vi "Configure Smoothing.vi"(7 "Enable Calculate1 (T: Enable)":bool=TRUE, 8 "error in (no error)":errorcluster, 9 "Enable Smoothing (T: Enable)":bool=TRUE, 10 "Measurement Number (2: Fast)":i32(ring)=2 items=["Slow", "Medium", "Fast"], 11 "VISA resource name":refnum<visa-resource-name>) -> (0 "error out":errorcluster, 3 "VISA resource name out":refnum<visa-resource-name>)   [LabVIEW 2021, in "Agilent 532XX Series.lvlib"]
doc: "Configures the parameters required for smoothing (moving average) filter on the measurements."
uses:
  <instrlib>/Agilent 532XX Series/Agilent 532XX Series.lvlib
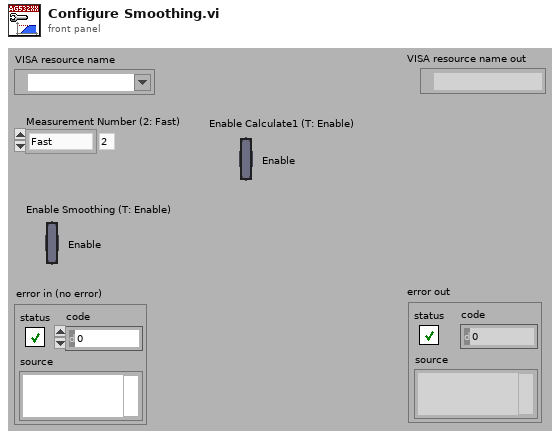
[diagram p1: front panel]
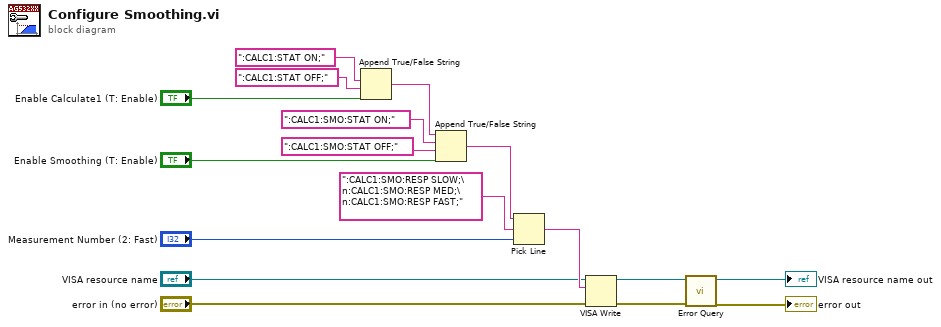
[diagram p0: block diagram]
diagram:
  n1 = Append True/False String(1:"Enable Calculate1 (T: Enable)", 2:":CALC1:STAT OFF;", 3:":CALC1:STAT ON;") -> (0:w14:string)  [unwired: 1 out]
  n2 = Append True/False String(1:"Enable Smoothing (T: Enable)", 2:":CALC1:SMO:STAT OFF;", 3:":CALC1:SMO:STAT ON;", 4:w14) -> (0:w10:string)
  n3 = Pick Line(string ("")=w10, multi-line string=":CALC1:SMO:RESP SLOW;\n:CALC1:SMO:RESP MED;\n:CALC1:SMO:RESP FAST;", line index="Measurement Number (2: Fast)") -> (output string=w9:string)
  n4 = VISA Write(VISA resource name="VISA resource name", write buffer=w9, error in (no error)="error in (no error)") -> (VISA resource name out=w6:refnum<visa-resource-name>, error out=w5:errorcluster)  [unwired: 1 out]
  n5 = call <instrlib>:"Error Query.vi"("error in (no error)"=w5, "VISA resource name"=w6) -> ("error out"=→"error out":errorcluster, "VISA resource name out"=→"VISA resource name out":refnum<visa-resource-name>)  [unwired: 8 out]
